vi "Find Center_01282025.vi"(5 "Position":i32, 7 "Tray Number":dbl format="%#_13g", 8 "Assembly Type":string, 9 "XYZTheta":dbl[](array[numeric]), 11 "Gantry In":refnum<k24>) -> (0 "Pedestal Height":dbl[](array[numeric]), 1 "XYZTheta Centers":dbl[][](array[numeric]), 3 "Gantry Out":refnum<k24>)   [LabVIEW 2021, in "Assembly Tray.lvclass"]
uses:
  Assembly Tray.lvclass
  Find Tray.ctl
  Controller/Camera/Machine Vision.ctl
  C:/Program Files (x86)/Aerotech/A3200/LabVIEW/2010/Bin/Aerotech.A3200.dll
  Program Files (x86)/Aerotech/A3200/LabVIEW/2010/Bin/Aerotech.A3200.dll
  Controller/Camera/Image processing.ctl
  Controller/Camera/Camera settings.ctl
  Controller/Camera/Material.ctl
  Controller/Camera/Camera.lvclass
  Controller/Motion/A3200/A3200.lvclass
  Controller/Motion/Motion.lvclass
panel:
  out "Low Speed":bool
  out "X":bool
  out "Y":bool
  out "Z":bool
  out "High Speed":bool
  out "Boolean 4":bool
  in  "Boolean 3":bool
  out "Move by":dbl[](array[numeric])
  in  "Autofiducial (Beta)":bool
  in  "Focus step size":dbl format="%#_13g"
  in  "number of focus steps":i32
  out "Average Strength":dbl
  in  "Focus":bool
  in  "Material":T1
  in  "Camera settings":T2={"Gamma"=1.6, "Gain"=0, "Sharpness"=0, "Contrast"=0.0, "Exposure"=0.0078125} {"Exposure" min=0.000244140625 max=0.5 scale=0.0002..0.5; "Contrast" min=0.0 max=1.0 scale=0.001..1.0; "Sharpness" min=0 max=2 step=1 scale=0.0..2.0; "Gain" min=0 max=100 step=1 scale=0.1..100.0; "Gamma" min=0.01 max=10.0 scale=0.01..10.0}
  in  "Image processing":T3={"Brightness"=128.0, "Contrast"=45.0, "Gamma"=1.0471123} {"Brightness" scale=0.0..400.0; "Contrast" scale=0.0..90.0; "Gamma" scale=0.005..5.0}
  in  "Override presets":bool
  out "Both fiducials recorded":bool
  in  "Machine Vision":T4
  out "Right Fiducial":dbl[](array[numeric]) format="%.6g"
  out "Left Fiducial":dbl[](array[numeric]) format="%.6g"
  out "Gantry":dbl[](array[numeric]) format="%.6g"
  out "Sum":dbl[](array[numeric]) format="%.6g"
  out "Camera":dbl[](array[numeric]) format="%.6g"
  in  "Carrier Tray":T5
  out "Image":T6(plugin-control)
  out "Center":dbl[](array[numeric]) format="%.6g"
  in  "Position Number":i16
  in  "Go to Center":bool
  in  "Calculate":bool
  in  "Record Bottom":bool
  in  "Record Top":bool
  in  "Go to Bottom Fiducial":bool
  in  "Go to Top Fiducial":bool
  in  "Joystick":bool
  in  "Stop":bool
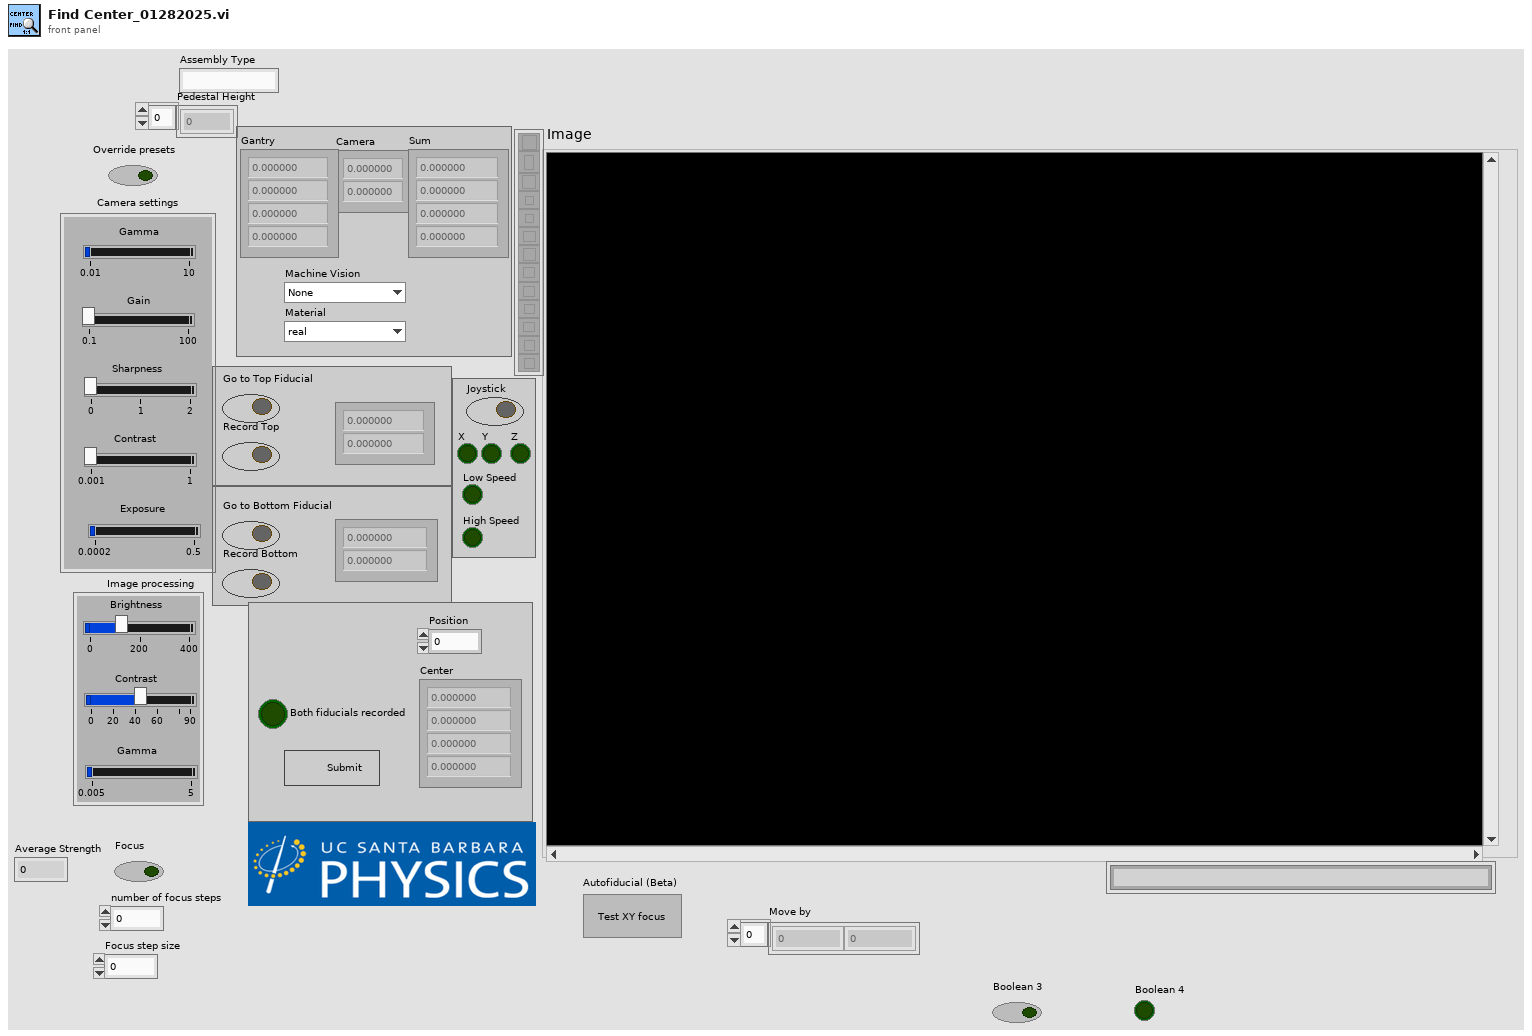
[diagram p1: front panel]
types:
  T1 = typedef "Camera.lvclass/Material.ctl" = enum16{"real", "dummy", "PETG"}
  T2 = typedef "Camera.lvclass/Camera settings.ctl" = cluster{"Gamma":dbl, "Gain":i64, "Sharpness":i64, "Contrast":dbl, "Exposure":dbl}
  T3 = typedef "Camera.lvclass/Image processing.ctl" = cluster{"Brightness":sgl, "Contrast":sgl, "Gamma":sgl}
  T4 = typedef "Camera.lvclass/Machine Vision.ctl" = enum16{"None", "Tray Fiducials", "V3 Sensor Circle", "Partial Hexaboard", "HPK Silicon", "Partial Hexaboard Test", "100um dot", "Hexaboard", "Corner (TL, BR)", "Corner (BL, TR)", "V3 Sensor Cross", "test", "Sensor Fiducials"}
  T5 = typedef "Assembly Tray.lvclass/Find Tray.ctl" = cluster{"Gantry Fiducials":dbl[], "Relative Coordinates":dbl[][], "Camera Fiducials":dbl[][], "XYZTheta Centers":dbl[][], "Workspace Center":dbl[], "Syringe Relative Coordinates":dbl[], "Gantry Region":dbl, "Fiducials":path, "New Fiducials":dbl[][], "Past Fiducials":dbl[][], "XYZTheta":dbl[], "Pedestal Height":dbl[]}
  T6 = typedef "IMAQ Image.ctl" = refnum<image>
  T7 = typedef "File Paths.ctl" = cluster{"Glue Pattern Folder":path, "Carrier Tray Folder":path, "Pick Up Tool Fixture Folder":path, "Components Folder":path, "Bellows Tool Offset.txt":path, "Pick Up Tool Offset.txt":path, "Dispense Tip Offset.txt":path, "Log Files":path, "Gantry Assembly Map.txt":path, "Syringe and offset map.txt":path, "Controllers Folder":path, "Local dbase config":path}
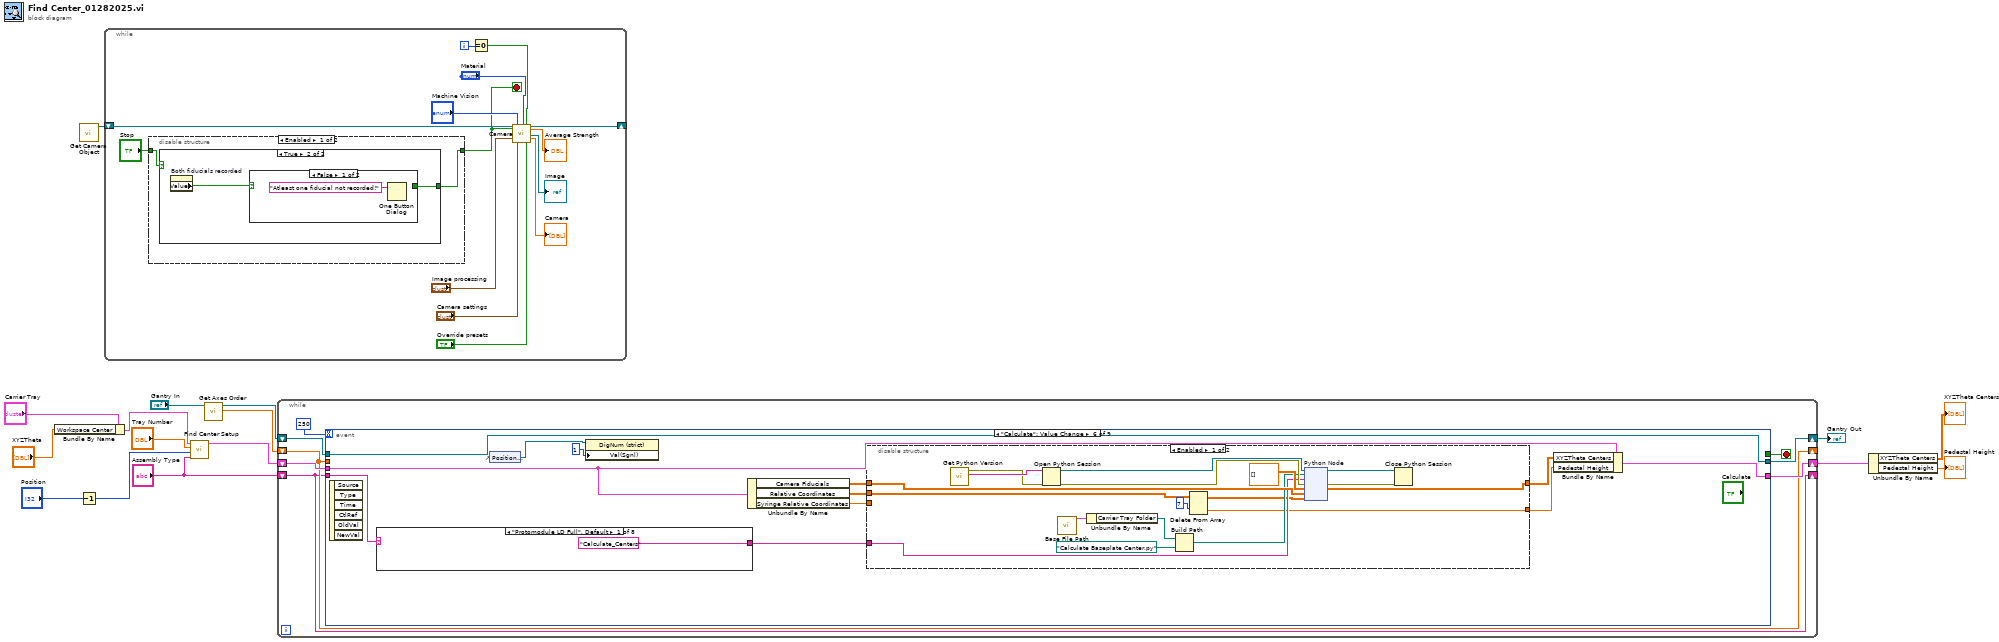
[diagram p0: block diagram]
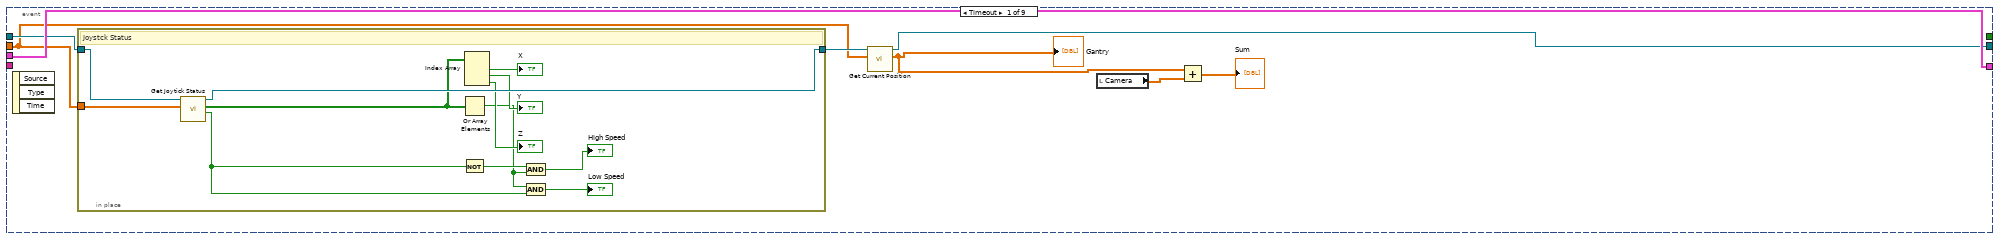
[diagram p2: hidden frame]
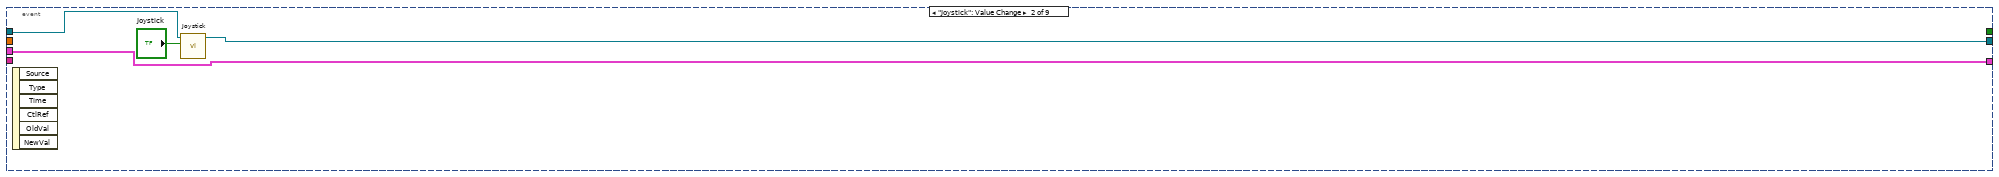
[diagram p3: hidden frame]
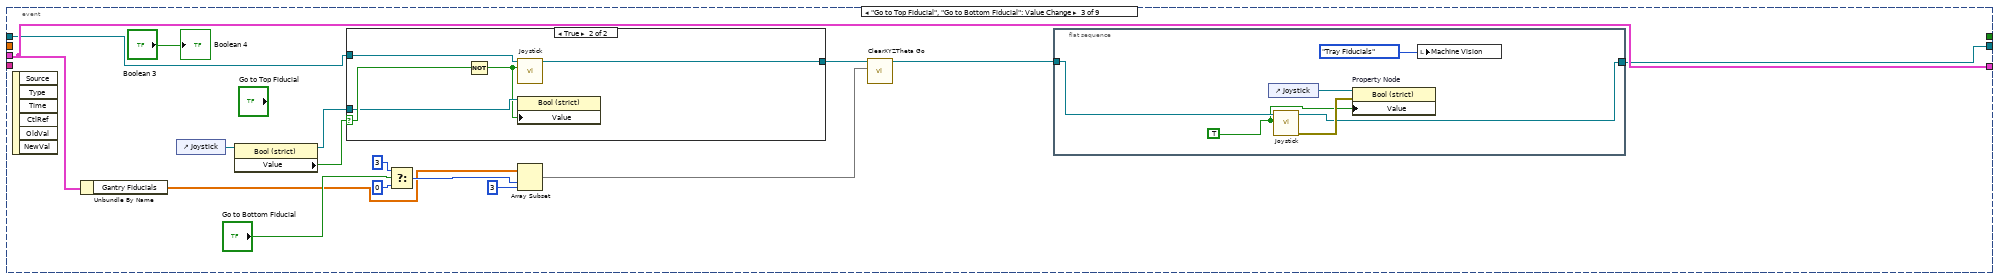
[diagram p4: hidden frame]
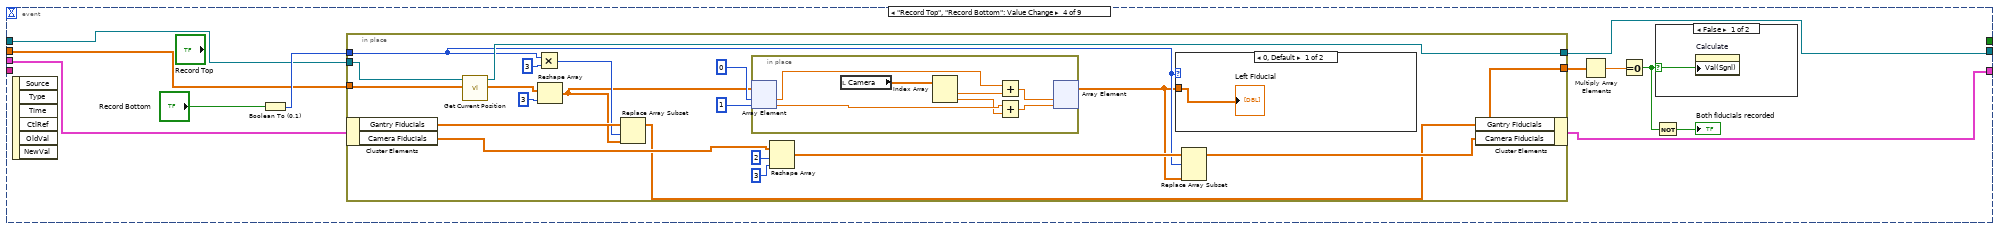
[diagram p6: hidden frame]
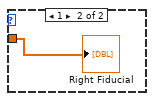
[diagram p8: hidden frame]
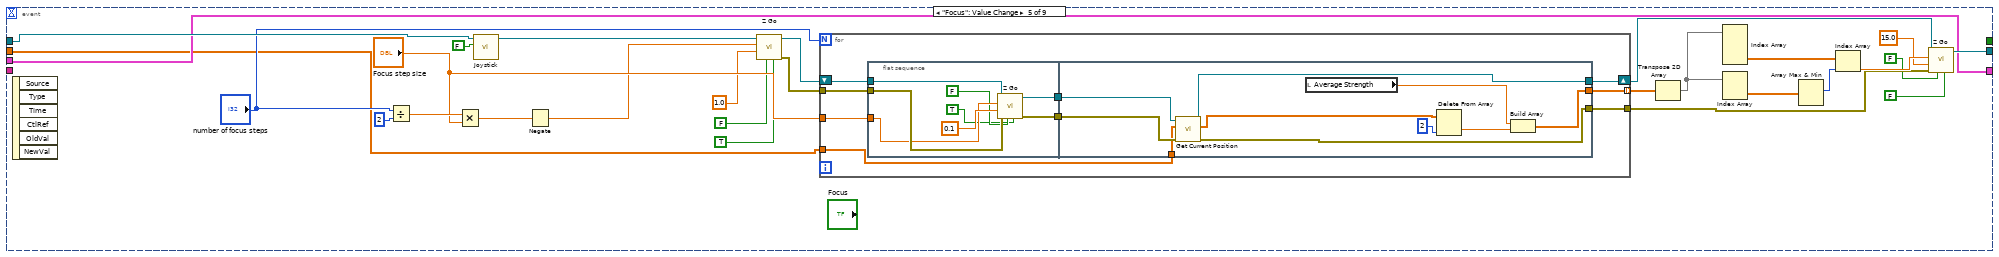
[diagram p9: hidden frame]
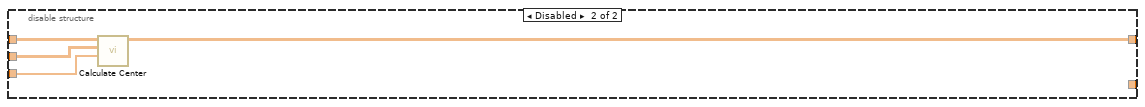
[diagram p10: hidden frame]
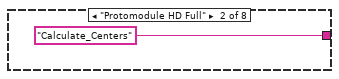
[diagram p11: hidden frame]
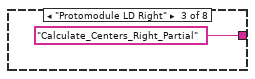
[diagram p12: hidden frame]
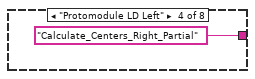
[diagram p13: hidden frame]
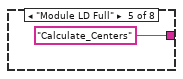
[diagram p14: hidden frame]
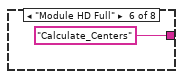
[diagram p15: hidden frame]
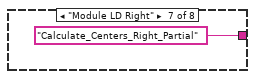
[diagram p16: hidden frame]
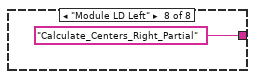
[diagram p17: hidden frame]
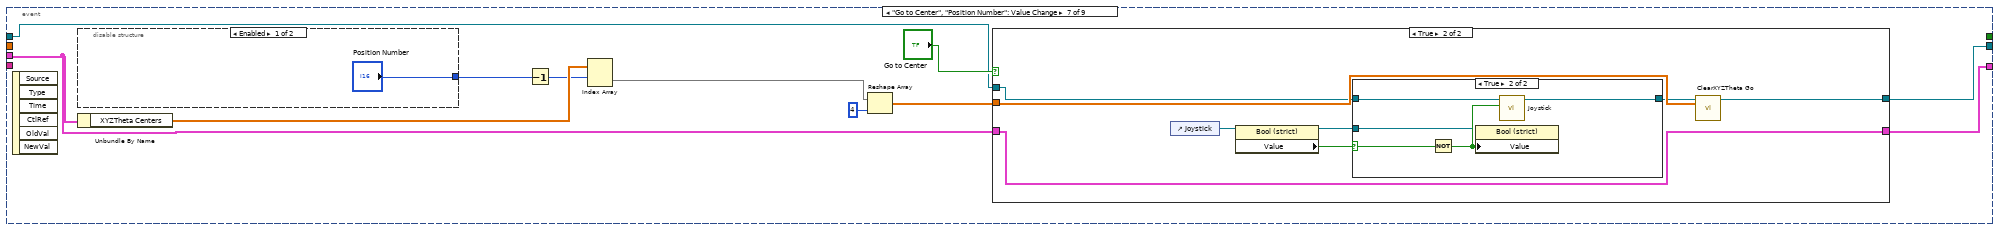
[diagram p18: hidden frame]
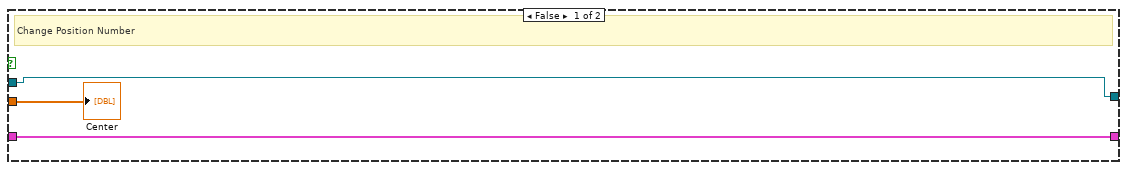
[diagram p20: hidden frame]
diagram:
  n1 = Bundle By Name(cluster="Carrier Tray", "Workspace Center"="XYZTheta") -> (w13:T5)
  n2 = call "Get Camera Object.vi"() -> ("Camera out"=w9:refnum<class "Camera.lvclass">)  [unwired: 10 in, 1 out]
  n3 = Decrement(x="Position") -> (x-1=w7:i32)
  n4 = while {
    shift-right: [w26] -> _
    shift-left: w9 -> [w30]
    i -> [w20]
    stop <- w25 stop-if-true
    n5 = disable-structure shown="Enabled" {
      disable-tunnel: [w31 w38] -> w25
      disable-tunnel: "Stop" -> [w32 w38]
      frame Enabled {
        n6 = case shown="True" w32 {
          tunnel: [_ w33] -> w31
          frame False {
          }
          frame True {
            n7 = property on="Both fiducials recorded" class="Bool (strict)"() -> ("Value"=w34:bool)  [unwired: 2 in, 2 out]
            n8 = case shown="False" w34 {
              tunnel: [_ TRUE] -> w33
              frame False {
                n9 = One Button Dialog(message="Atleast one fiducial not recorded!") -> ()  [unwired: 1 in, 1 out]
              }
              frame True {
                n10 = property on="Both fiducials recorded" class="Bool (strict)"("Val(Sgnl)"=FALSE) -> ()  [unwired: 2 in, 2 out]
              }
            }
          }
        }
      }
      frame Disabled {
      }
    }
    n11 = Equal To 0?(x=w20) -> (x = 0?=w19:bool)
    n12 = call "Camera.vi"("Camera in"=w30, "Stop"=w25, "BCG Image Processing"="Image processing", "Machine Vision"="Machine Vision", "Camera settings"="Camera settings", "Material"="Material", "Loop 0"=w19, "Override presets"="Override presets") -> ("Camera out"=w26:refnum<class "Camera.lvclass">, "Average Strength"=→"Average Strength":dbl, "Image"=→"Image":T6, "Camera"=→"Camera":dbl[])  [unwired: 5 in, 3 out]
  }
  n13 = call "Find Center Setup.vi"("Carrier Tray"=w13, "Tray Number"="Tray Number", "Position"=w7, "Assembly Type"="Assembly Type") -> ("Assembly Tray Out"=w16:T5)  [unwired: 6 in]
  n14 = call "Get Axes Order.vi"("Gantry In"="Gantry In") -> ("Axes Order"=w3:dbl[], "Gantry Out"=w4:refnum<k24>)  [unwired: 8 in, 1 out]
  n15 = while {
    shift-right: [w45] -> w15
    shift-left: w16 -> [w46]
    shift-right: [w41] -> w8
    shift-left: w4 -> [w42]
    shift-right: [w40] -> _
    shift-left: w3 -> [w40]
    shift-right: [w39] -> _
    shift-left: "Assembly Type" -> [w39]
    stop <- w44 stop-if-true
    n16 = event shown="[5] \"Calculate\": Value Change" {
      selector: _ -> [_ _ _ _ _ _ _ _ _]
      dyn-events: _ -> [_ _ _ _ _ _ _ _ _]
      timeout: 250 -> [_ _ _ _ _ _ _ _ _]
      tunnel: [w52 w70 w86 w109 w151 w197 w245 w272 w285] -> w45
      tunnel: w46 -> [w52 w70 w86 w104 w151 w198 w246 w272 w285]
      tunnel: [_ _ _ _ _ _ _ w267 _] -> w44
      tunnel: w42 -> [w49 w69 w78 w103 w153 w203 w243 w273 w287]
      tunnel: [w50 w67 w73 w102 w152 w203 w240 w268 w288] -> w41
      tunnel: w39 -> [_ _ _ _ _ w199 _ _ _]
      tunnel: w40 -> [w47 _ _ w99 w139 _ _ _ _]
      event Timeout {
        n17 = event-data() -> ()  [unwired: 1 in, 3 out]
        n18 = in-place {
          in-place-border: w49 -> [w66]
          in-place-border: [w65] -> w48
          in-place-border: w47 -> [w64]
          # "Joystck Status"
          n19 = call "Get Joytick Status.vi"("Axes Order"=w64, "Gantry In"=w66) -> ("JoystickLowSpeedActive"=w58:bool, "Joystick Status"=w60:bool[], "Gantry Out"=w65:refnum<k24>)  [unwired: 6 in, 1 out]
          n20 = Or Array Elements(Boolean array=w60) -> (logical OR=w56:bool)
          n21 = Not(x=w58) -> (.not. x?=w57:bool)
          n22 = Index Array(array=w60) -> (element #1=→"X":bool, element #2=→"Y":bool, element #3=→"Z":bool)  [unwired: 3 in]
          n23 = And(x=w57, y=w56) -> (x .and. y?=→"High Speed":bool)
          n24 = And(x=w56, y=w58) -> (x .and. y?=→"Low Speed":bool)
        }
        n25 = call "Get Current Position.vi"("Axes Order"=w47, "Gantry In"=w48) -> ("XYZTheta Out"=w51:dbl[], "Gantry Out"=w50:refnum<k24>)  [unwired: 7 in, 1 out]
        "Gantry" <- w51
        n26 = local read "Camera"() -> (w54:dbl[])
        n27 = Add(x=w51, y=w54) -> (x+y=→"Sum":dbl[])
      }
      event "Joystick": Value Change {
        n28 = event-data() -> ()  [unwired: 1 in, 6 out]
        n29 = call "Joystick.vi"("Joystick"="Joystick", "Gantry In"=w69) -> ("Gantry Out"=w67:refnum<k24>)  [unwired: 8 in, 1 out]
      }
      event "Go to Top Fiducial", "Go to Bottom Fiducial": Value Change {
        n30 = event-data() -> ()  [unwired: 1 in, 6 out]
        n31 = Unbundle By Name "Unbundle By Name"(w86) -> ("Gantry Fiducials"=w75:dbl[])
        n32 = control-ref of="Joystick"() -> (w85:refnum<vi>)
        n33 = property class="Bool (strict)"(reference=w85) -> (reference out=w76:refnum<vi>, "Value"=w79:bool)  [unwired: 1 in, 1 out]
        n34 = case shown="True" w79 {
          selector: w79 -> [_ w98]
          tunnel: w78 -> [w93 w96]
          tunnel: [w93 w95] -> w77
          tunnel: w76 -> [_ w97]
          frame False {
          }
          frame True {
            n35 = Not(x=w98) -> (.not. x?=w94:bool)
            n36 = call "Joystick.vi"("Joystick"=w94, "Gantry In"=w96) -> ("Gantry Out"=w95:refnum<k24>)  [unwired: 8 in, 1 out]
            n37 = property class="Bool (strict)"(reference=w97, "Value"=w94) -> ()  [unwired: 1 in, 2 out]
          }
        }
        n38 = Select(t=3, s="Go to Bottom Fiducial", f=0) -> (s? t:f=w83:i32)
        n39 = Array Subset "Array Subset"(array=w75, index=w83, length=3) -> (w74:dbl[])
        n40 = call "ClearXYZTheta Go.vi"("XYZTheta In"=w74, "Gantry In"=w77) -> ("Gantry Out"=w72:refnum<k24>)  [unwired: 7 in, 2 out]
        n41 = flat-sequence {
          tunnel: w72 -> [w92]
          tunnel: [w89] -> w73
          frame #0 {
            w88 = TRUE
            n42 = control-ref of="Joystick"() -> (w91:refnum<vi>)
            n43 = call "Joystick.vi"("Joystick"=w88, "Gantry In"=w92) -> ("error out"=w90:errorcluster, "Gantry Out"=w89:refnum<k24>)  [unwired: 8 in]
            n44 = property on="Property Node" class="Bool (strict)"(reference=w91, error in=w90, "Value"=w88) -> ()  [unwired: 2 out]
            n45 = local write "Machine Vision"(Machine_Vision."Tray Fiducials" ("Machine Vision")) -> ()
          }
        }
        "Boolean 4" <- "Boolean 3"
      }
      event "Record Top", "Record Bottom": Value Change {
        n46 = event-data() -> ()  [unwired: 1 in, 6 out]
        n47 = Boolean To (0,1)(Boolean="Record Bottom") -> (0, 1=w106:i16)
        n48 = in-place {
          in-place-border: [w123] -> w107
          in-place-border: w106 -> [w116]
          in-place-border: w103 -> [w118]
          in-place-border: [w117] -> w102
          in-place-border: w99 -> [w111]
          n49 = in-place-cluster #1(w104) -> ("Gantry Fiducials"=w120:dbl[], "Camera Fiducials"=w127:dbl[][])
          n50 = call "Get Current Position.vi"("Axes Order"=w111, "Gantry In"=w118) -> ("XYZTheta Out"=w121:dbl[], "Gantry Out"=w117:refnum<k24>)  [unwired: 7 in, 1 out]
          n51 = Multiply(x=w116, y=i16 3) -> (x*y=w114:i16)
          n52 = Reshape Array(w121, 3 ("dimension size")) -> (w113:dbl[])
          n53 = Replace Array Subset(array=w120, new element=w113, index=w114) -> (w119:dbl[])
          n54 = in-place {
            n55 = in-place-array #2(w113, 0, 1) -> (w135:dbl, w133:dbl)
            n56 = local read "Camera"() -> (w136:dbl[])
            n57 = Index Array(array=w136) -> (element #1=w134:dbl, element #2=w132:dbl)  [unwired: 2 in]
            n58 = Add(x=w135, y=w134) -> (x+y=w130:dbl)
            n59 = Add(x=w133, y=w132) -> (x+y=w131:dbl)
            n60 = in-place-array #2(w130, w131) -> (w112:dbl[])  [unwired: 2 out]
          }
          n61 = Reshape Array(w127, 2 ("length"), 3 ("dimension size")) -> (w126:dbl[][])
          n62 = case shown="0, Default" w116 {
            tunnel: w112 -> [w137 w138]
            frame 0, Default {
              "Left Fiducial" <- w137
            }
            frame 1 {
              "Right Fiducial" <- w138
            }
          }
          n63 = Replace Array Subset(array=w126, new element=w112, index (row)=w116) -> (w123:dbl[][])  [unwired: 1 in]
          n64 = in-place-cluster #1("Gantry Fiducials"=w119, "Camera Fiducials"=w123) -> (w109:T5)
        }
        n65 = Multiply Array Elements(1:w107) -> (0:w108:dbl)
        n66 = Equal To 0?(x=w108) -> (x = 0?=w101:bool)
        n67 = Not(x=w101) -> (.not. x?=→"Both fiducials recorded":bool)
        n68 = case shown="False" w101 {
          selector: w101 -> [w110 _]
          frame False {
            n69 = property on="Calculate" class="Bool (strict)"("Val(Sgnl)"=w110) -> ()  [unwired: 2 in, 2 out]
          }
          frame True {
          }
        }
      }
      event "Focus": Value Change {
        n70 = event-data() -> ()  [unwired: 1 in, 6 out]
        n71 = Divide(x="number of focus steps", y=2) -> (x/y=w155:dbl)
        n72 = Multiply(x=w155, y="Focus step size") -> (x*y=w154:dbl)
        n73 = call "Joystick.vi"("Joystick"=FALSE, "Gantry In"=w153) -> ("Gantry Out"=w147:refnum<k24>)  [unwired: 8 in, 1 out]
        n74 = Negate(x=w154) -> (-x=w145:dbl)
        n75 = call "Z Go.vi"("Increment"=TRUE, "Return Immediately"=FALSE ("Increment"), "Speed In"=1.0 ("Speed"), "Position In"=w145, "Gantry In"=w147) -> ("error out"=w142:errorcluster, "Gantry Out"=w146:refnum<k24>)  [unwired: 3 in, 2 out]
        n76 = for {
          N: "number of focus steps" -> [_]
          tunnel: [w172] -> w165 mode=indexing
          tunnel: w142 -> [w171]
          tunnel: [w169] -> w158
          shift-right: [w173] -> w159
          shift-left: w146 -> [w175]
          tunnel: "Focus step size" -> [w168]
          tunnel: w139 -> [w167]
          n77 = flat-sequence {
            tunnel: w175 -> [w183]
            tunnel: [w182] -> w174
            tunnel: w171 -> [w180]
            tunnel: [w181] -> w170
            tunnel: w168 -> [w178]
            tunnel: w174 -> [w193]
            tunnel: [w192] -> w173
            tunnel: [w191] -> w172
            tunnel: w170 -> [w187]
            tunnel: [w186] -> w169
            tunnel: w167 -> [w184]
            frame #0 {
              n78 = call "Z Go.vi"("Increment"=TRUE, "Return Immediately"=FALSE ("Increment"), "error in (no error)"=w180, "Speed In"=0.1 ("Speed"), "Position In"=w178, "Gantry In"=w183) -> ("error out"=w181:errorcluster, "Gantry Out"=w182:refnum<k24>)  [unwired: 2 in, 2 out]
            }
            frame #1 {
              n79 = call "Get Current Position.vi"("error in (no error)"=w187, "Axes Order"=w184, "Gantry In"=w193) -> ("error out"=w186:errorcluster, "XYZTheta Out"=w190:dbl[], "Gantry Out"=w192:refnum<k24>)  [unwired: 6 in]
              n80 = local read "Average Strength"() -> (w185:dbl)
              n81 = Delete From Array(array=w190, index=2) -> (deleted portion=w188:dbl)  [unwired: 1 in, 1 out]
              n82 = Build Array(w185, w188) -> (w191:dbl[])
            }
          }
        }
        n83 = Transpose 2D Array(2D array=w165) -> (transposed array=w164:dbl[][])
        n84 = Index Array(array=w164) -> (element #2=w163:dbl[])  [unwired: 4 in, 1 out]
        n85 = Index Array(array=w164) -> (element=w166:dbl[])  [unwired: 2 in]
        n86 = Array Max & Min(array=w166) -> (max index (indices)=w162:i32)  [unwired: 3 out]
        n87 = Index Array(array=w163, index=w162) -> (element=w161:dbl)
        n88 = call "Z Go.vi"("Increment"=FALSE, "Return Immediately"=FALSE ("Increment"), "error in (no error)"=w158, "Speed In"=15.0 ("Speed"), "Position In"=w161, "Gantry In"=w159) -> ("Gantry Out"=w152:refnum<k24>)  [unwired: 2 in, 3 out]
      }
      event "Calculate": Value Change {
        n89 = event-data() -> ()  [unwired: 1 in, 6 out]
        n90 = case shown="\"Protomodule LD Full\", Default" w199 {
          tunnel: ["Calculate_Centers" ("function name") "Calculate_Centers" ("function name") "Calculate_Centers_Right_Partial" ("function name") "Calculate_Centers_Right_Partial" ("function name") "Calculate_Centers" ("function name") "Calculate_Centers" ("function name") "Calculate_Centers_Right_Partial" ("function name") "Calculate_Centers_Right_Partial" ("function name")] -> w196
          frame "Protomodule LD Full", Default {
          }
          frame "Protomodule HD Full" {
          }
          frame "Protomodule LD Right" {
          }
          frame "Protomodule LD Left" {
          }
          frame "Module LD Full" {
          }
          frame "Module HD Full" {
          }
          frame "Module LD Right" {
          }
          frame "Module LD Left" {
          }
        }
        n91 = control-ref of="Position Number"() -> (w205:refnum<vi>)
        n92 = property class="DigNum (strict)"(reference=w205, "Val(Sgnl)"=i16 1 ("Value (Signaling)")) -> ()  [unwired: 1 in, 2 out]
        n93 = Unbundle By Name "Unbundle By Name"(w198) -> ("Camera Fiducials"=w200:dbl[][], "Relative Coordinates"=w201:dbl[][], "Syringe Relative Coordinates"=w202:dbl[])
        n94 = disable-structure shown="Enabled" {
          disable-tunnel: w200 -> [w218 w226]
          disable-tunnel: w201 -> [w209 w225]
          disable-tunnel: w202 -> [_ w224]
          disable-tunnel: [w213 w227] -> w195
          disable-tunnel: w196 -> [w212 _]
          disable-tunnel: [w206 _] -> w194
          frame Enabled {
            n95 = call "Get Python Version.vi"() -> ("Python Version"=w211:string, "error out"=w210:errorcluster)  [unwired: 10 in]
            n96 = Open Python Session(python version=w211, 3:w210) -> (session out=w223:refnum<k35>, error out=w221:errorcluster)  [unwired: 1 in]
            n97 = call "Base File Path.vi"() -> ("Paths Out"=w219:T7)  [unwired: 11 in]
            n98 = Unbundle By Name(w219) -> ("Carrier Tray Folder"=w216:path)
            n99 = Build Path(base path=w216, name or relative path=path "Calculate Baseplate Center.py") -> (appended path=w215:path)
            n100 = Delete From Array(array=w209, index (row)=7) -> (deleted portion=w206:dbl[], array with subset deleted=w207:dbl[][])  [unwired: 2 in]
            n101 = node "Python Node"(w223, w215, w212, w221, dbl[][] [], w218, w207) -> (w222:refnum<k35>, w220:errorcluster, w213:dbl[][])  [unwired: 2 in, 2 out]
            n102 = Close Python Session(session in=w222, error in=w220) -> ()  [unwired: 1 out]
          }
          frame Disabled {
            n103 = call "Calculate Center.vi"("Syringe Coordinates"=w224, "Relative Coordinates"=w225, "Fiducial Measurements"=w226) -> ("XYZTheta Centers"=w227:dbl[][])  [unwired: 8 in]
          }
        }
        n104 = Bundle By Name(cluster=w198, "XYZTheta Centers"=w195, "Pedestal Height"=w194) -> (w197:T5)
      }
      event "Go to Center", "Position Number": Value Change {
        n105 = event-data() -> ()  [unwired: 1 in, 6 out]
        n106 = disable-structure shown="Enabled" {
          disable-tunnel: ["Position Number" _] -> w237
          frame Enabled {
          }
          frame Disabled {
          }
        }
        n107 = Unbundle By Name(w246) -> ("XYZTheta Centers"=w239:dbl[][])
        n108 = Decrement(x=w237) -> (x-1=w238:i16)
        n109 = Index Array "Index Array"(array=w239, index (row)=w238) -> (element=w241:dbl[])  [unwired: 1 in]
        n110 = Reshape Array "Reshape Array"(w241, u32 4) -> (w236:dbl[])
        n111 = case shown="True" "Go to Center" {
          tunnel: w236 -> [w248 w256]
          tunnel: w246 -> [w250 w258]
          tunnel: [w250 w258] -> w245
          tunnel: w243 -> [w249 w252]
          tunnel: [w249 w257] -> w240
          frame False {
            # "Change Position Number"
            "Center" <- w248
          }
          frame True {
            n112 = control-ref of="Joystick"() -> (w255:refnum<vi>)
            n113 = property class="Bool (strict)"(reference=w255) -> (reference out=w253:refnum<vi>, "Value"=w254:bool)  [unwired: 1 in, 1 out]
            n114 = case shown="True" w254 {
              selector: w254 -> [_ w264]
              tunnel: w252 -> [w259 w263]
              tunnel: [w259 w262] -> w251
              tunnel: w253 -> [_ w260]
              frame False {
              }
              frame True {
                n115 = Not(x=w264) -> (.not. x?=w261:bool)
                n116 = property class="Bool (strict)"(reference=w260, "Value"=w261) -> ()  [unwired: 1 in, 2 out]
                n117 = call "Joystick.vi"("Joystick"=w261, "Gantry In"=w263) -> ("Gantry Out"=w262:refnum<k24>)  [unwired: 8 in, 1 out]
              }
            }
            n118 = call "ClearXYZTheta Go.vi"("XYZTheta In"=w256, "Gantry In"=w251) -> ("Gantry Out"=w257:refnum<k24>)  [unwired: 7 in, 2 out]
          }
        }
      }
      event "Stop": Value Change {
        n119 = event-data() -> ()  [unwired: 1 in, 6 out]
        n120 = Unbundle By Name(w272) -> ("Fiducials"=w270:path, "Gantry Fiducials"=w271:dbl[])
        n121 = call "Replace Row In File.vi"("Index"=0, "Insert Array"=w271, "Path"=w270) -> ("error out"=w276:errorcluster)  [unwired: 8 in]
        n122 = property on="Both fiducials recorded" class="Bool (strict)"() -> ("Value"=w265:bool)  [unwired: 2 in, 2 out]
        n123 = case shown="No Error" w276 {
          tunnel: "Fiducial" -> [w277 w284]
          frame No Error {
            w278 = "\r"
            n124 = Concatenate Strings("Success!", w278, w278, w277, " Values Stored") -> ()  [unwired: 1 out]
          }
          frame Error {
            w281 = "\r"
            n125 = Concatenate Strings("Error!", w281, w281, w284, " Values Not Stored") -> ()  [unwired: 1 out]
          }
        }
        n126 = And(x=w265, y=TRUE) -> (x .and. y?=w267:bool)
        n127 = call "Joystick.vi"("Joystick"=FALSE, "Gantry In"=w273) -> ("Gantry Out"=w268:refnum<k24>)  [unwired: 8 in, 1 out]
      }
      event "Autofiducial (Beta)": Value Change {
        n128 = event-data() -> ()  [unwired: 1 in, 6 out]
        n129 = disable-structure shown="Enabled" {
          disable-tunnel: [w292 w319] -> w288
          disable-tunnel: w287 -> [w291 w319]
          disable-tunnel: "Autofiducial (Beta)" -> [w290 _]
          frame Enabled {
            n130 = flat-sequence {
              tunnel: w290 -> [_]
              tunnel: [w298] -> w289
              tunnel: w291 -> [w303]
              tunnel: [w303] -> w297
              tunnel: [w302] -> w296
              tunnel: [w301] -> w295
              tunnel: w289 -> [w300]
              tunnel: w297 -> [w307]
              tunnel: [w306] -> w294
              tunnel: w296 -> [w305]
              tunnel: [w304] -> w293
              tunnel: w295 -> [w304]
              tunnel: [w313] -> w292
              tunnel: w294 -> [w314]
              tunnel: w293 -> [w312]
              frame #0 {
                n131 = local read "Image"() -> (w299:T6)
                n132 = call "Find Fiducial.vi"("Image"=w299) -> ("Move by (mm)"=w298:dbl[])  [unwired: 3 in]
              }
              frame #1 {
                n133 = Index Array(array=w300) -> (element #1=w302:dbl, element #2=w301:dbl)  [unwired: 2 in]
                "Move by" <- w300
              }
              frame #2 {
                n134 = call "Joystick.vi"("Joystick"=FALSE, "Gantry In"=w307) -> ("Gantry Out"=w308:refnum<k24>)  [unwired: 8 in, 1 out]
                n135 = call "Move Inc.vi"("Axis"="X", "Speed"=1.0, "Distance"=w305, "Gantry In"=w308) -> ("Gantry Out"=w306:refnum<k24>)  [unwired: 6 in, 1 out]
              }
              frame #3 {
                n136 = call "Joystick.vi"("Joystick"=FALSE, "Gantry In"=w314) -> ("Gantry Out"=w315:refnum<k24>)  [unwired: 8 in, 1 out]
                n137 = call "Move Inc.vi"("Axis"="Y", "Speed"=1.0, "Distance"=w312, "Gantry In"=w315) -> ("Gantry Out"=w313:refnum<k24>)  [unwired: 6 in, 1 out]
              }
            }
          }
          frame Disabled {
          }
        }
      }
    }
  }
  "Gantry Out" <- w8
  n138 = Unbundle By Name(w15) -> ("XYZTheta Centers"=→"XYZTheta Centers":dbl[][], "Pedestal Height"=→"Pedestal Height":dbl[])
